vi "Query Sequence Completed Repetitions.vi"(8 "error in (no error)":errorcluster, 10 "Instance (1)":i32=1, 11 "VISA resource name":refnum<visa-resource-name>) -> (0 "error out":errorcluster, 2 "Repetitions":i32, 3 "VISA resource name out":refnum<visa-resource-name>)   [LabVIEW 2015, in "Rohde&Schwarz CMXP GPRF.lvlib"]
doc: "Queries the number of completed repetitions of the sequencer list, for repetition mode SINGle.\n\nAttribute(s):\nRSCMXPGPRF_ATTR_SEQUENCE_COMPLETED_REPETITIONS\n\nRemote-control command(s):\nSOURce:GPRF:GEN<i>:SEQuencer:RCOunt?"
uses:
  <instrlib>/Rohde&Schwarz CMXP GPRF/Rohde&Schwarz CMXP GPRF.lvlib
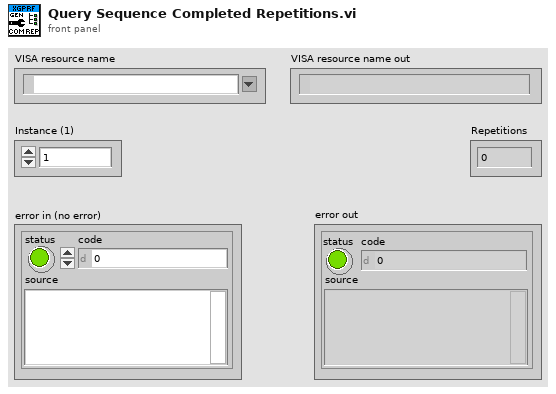
[diagram p1: front panel]
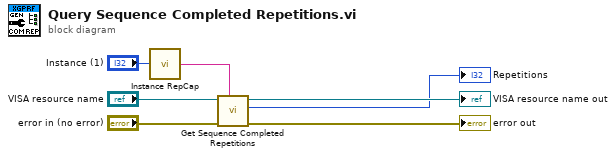
[diagram p0: block diagram]
diagram:
  n1 = call <instrlib>:"Instance RepCap.vi"("instance  in"="Instance (1)") -> ("instance out"=w3:string)
  n2 = call "Get Sequence Completed Repetitions"("Repeated Capabilities"=w3, "error in (no error)"="error in (no error)", "instrument handle"="VISA resource name") -> ("error out"=→"error out":errorcluster, "Sequence Completed Repetitions"=→"Repetitions":i32, "instrument handle out"=→"VISA resource name out":refnum<visa-resource-name>)  [unwired: 6 in]
